vi "Set_Joint_Main_Loop.vi"(0 "X-CAN in":refnum<class "X-CAN.lvclass">, 1 "Actual position":T1(array[cluster]) {"Error Code" format="%b"; "ID" format="%x"}, 2 "Motor enabled?":bool[](array[boolean]), 5 "Reset?":bool[](array[boolean]), 7 "Desired position":u16[](array[numeric]) format="%x", 9 "Current position":u16[](array[numeric]) format="%x", 11 "error in (no error)":errorcluster, 12 "Speed":u16[](array[numeric]) format="%x", 13 "Reset speed?":bool) -> (4 "X-CAN out":refnum<class "X-CAN.lvclass">, 6 "New position":T1(array[cluster]) {"Error Code" format="%b"; "ID" format="%x"}, 15 "error out":errorcluster)   [LabVIEW 2015]
uses:
  <vilib>/Stratom, Inc/X-CAN for myRIO (API)/X-CAN Class/X-CAN.lvclass
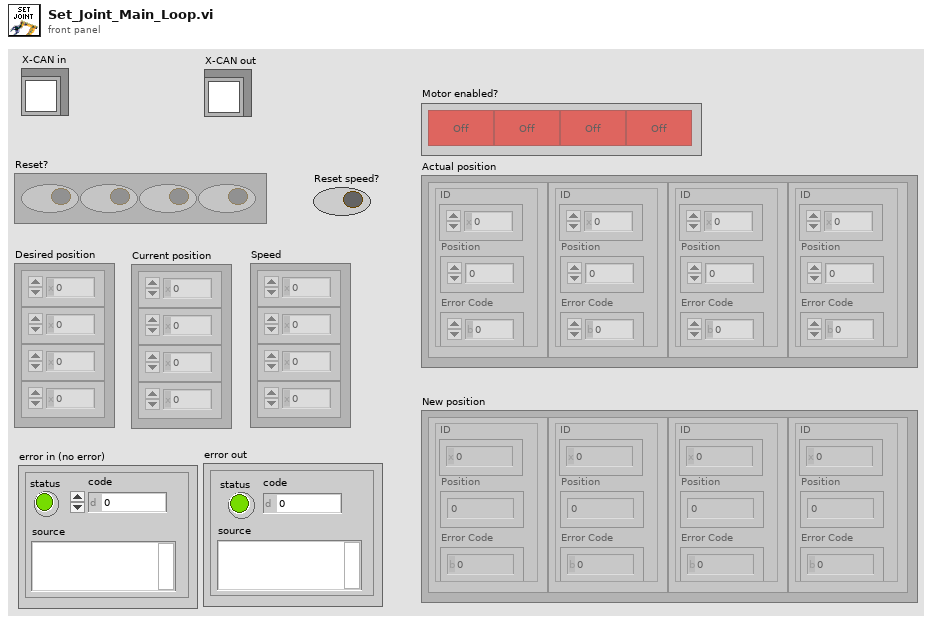
[diagram p1: front panel]
types:
  T1 = cluster{"ID":u8, "Position":u16, "Error Code":u8}[]
  T2 = typedef "X-CAN.lvclass/CANFrame.ctl" = cluster{"identifier":u32, "extended?":bool, "echo?":bool, "payload":u8[], "timestamp":timestamp}
  T3 = cluster{"Error Code":u8, "Position":u16, "ID":u8}
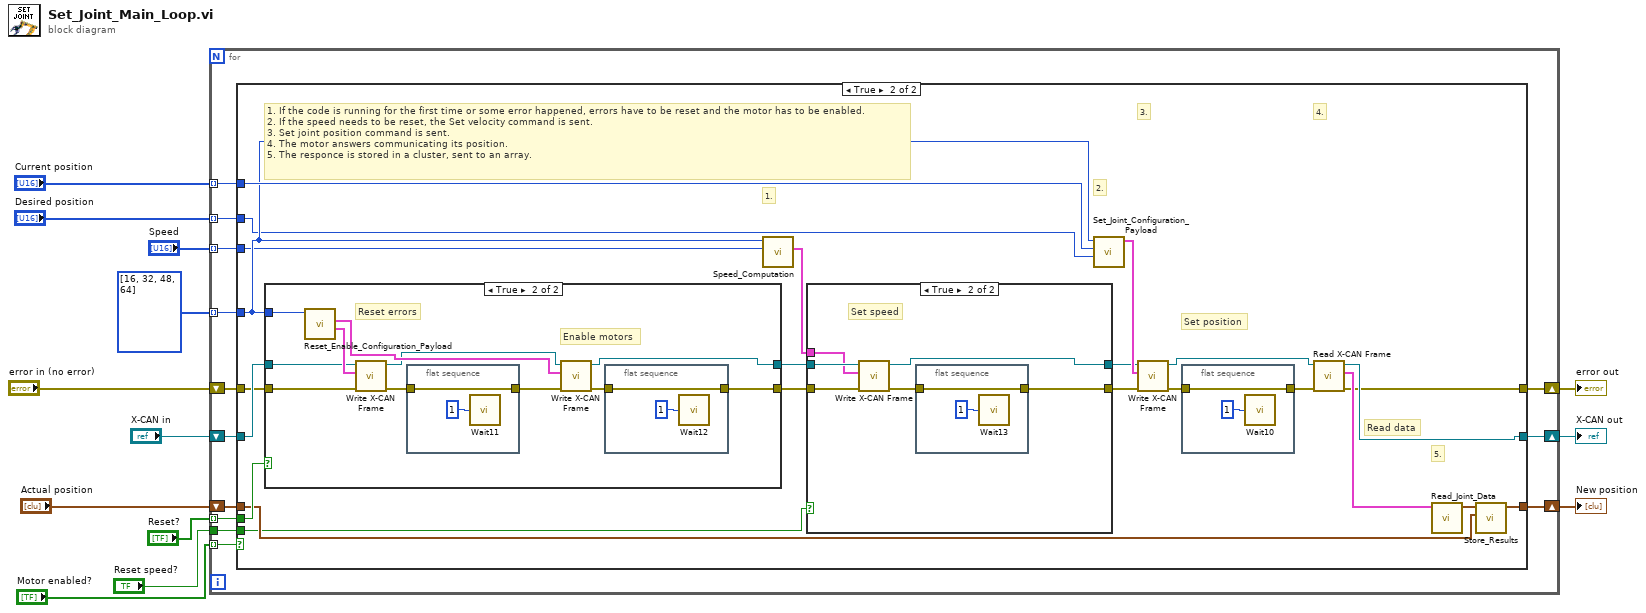
[diagram p0: block diagram]
diagram:
  n1 = for {
    shift-right: [w21] -> w10
    shift-left: "X-CAN in" -> [w26]
    shift-right: [w16] -> w11
    shift-left: "error in (no error)" -> [w25]
    tunnel: u8[] [16, 32, 48, 64] ("identifier") -> [w18] mode=indexing
    tunnel: "Reset?" -> [w24] mode=indexing
    tunnel: "Current position" -> [w20] mode=indexing
    tunnel: "Desired position" -> [w19] mode=indexing
    shift-right: [w23] -> w4
    shift-left: "Actual position" -> [w22]
    tunnel: "Speed" -> [w17] mode=indexing
    tunnel: "Motor enabled?" -> [w15] mode=indexing
    tunnel: "Reset speed?" -> [w14]
    n2 = case shown="True" w15 {
      tunnel: w26 -> [w28 w50]
      tunnel: w25 -> [w29 w49]
      tunnel: w24 -> [_ w48]
      tunnel: [w27 w47] -> w23
      tunnel: w22 -> [w27 w46]
      tunnel: [w28 w42] -> w21
      tunnel: w20 -> [_ w40]
      tunnel: w19 -> [_ w31]
      tunnel: w18 -> [_ w39]
      tunnel: w17 -> [_ w38]
      tunnel: [w29 w32] -> w16
      tunnel: w14 -> [_ w30]
      frame False {
      }
      frame True {
        # "1. If the code is running for the first time or some error happened, errors have to be reset and the motor has to be enabled.\n2. If the speed needs to be reset, the Set velocity command is sent.\n3. Set joint position command is sent.\n4. The motor answers communicating its position.\n5. The responce is stored in a cluster, sent to an array."
        # "5."
        # "4."
        # "3."
        # "2."
        # "1."
        # "Read data"
        # "Set position"
        n3 = case shown="True" w48 {
          tunnel: [w64 w69] -> w37
          tunnel: [w63 w68] -> w36
          tunnel: w50 -> [w64 w67]
          tunnel: w49 -> [w63 w66]
          tunnel: w39 -> [_ w65]
          frame False {
          }
          frame True {
            # "Enable motors"
            # "Reset errors"
            n4 = call "Reset_Enable_Configuration_Payload.vi"("identifier selection in"=w65) -> ("Reset errors command"=w71:T2, "Enable motor command"=w72:T2)  [unwired: 9 in]
            n5 = call <vilib>:"Write X-CAN Frame.vi"("error in"=w66, "CAN Frame"=w71, "X-CAN Session in"=w67) -> ("error out"=w73:errorcluster, "X-CAN Session out"=w70:refnum<class "X-CAN.lvclass">)  [unwired: 7 in]
            n6 = flat-sequence {
              tunnel: w73 -> [w78]
              tunnel: [w78] -> w75
              frame #0 {
                n7 = call "Wait11"("Count(mSec)"=u32 1 ("Tick Count(mSec)")) -> ()  [unwired: 1 out]
              }
            }
            n8 = call <vilib>:"Write X-CAN Frame.vi"("error in"=w75, "CAN Frame"=w72, "X-CAN Session in"=w70) -> ("error out"=w74:errorcluster, "X-CAN Session out"=w69:refnum<class "X-CAN.lvclass">)  [unwired: 7 in]
            n9 = flat-sequence {
              tunnel: w74 -> [w76]
              tunnel: [w76] -> w68
              frame #0 {
                n10 = call "Wait12"("Count(mSec)"=u32 1 ("Tick Count(mSec)")) -> ()  [unwired: 1 out]
              }
            }
          }
        }
        n11 = call "Speed_Computation.vi"("Speed"=w38, "identifier"=w39) -> ("output cluster"=w33:T2)  [unwired: 9 in]
        n12 = case shown="True" w30 {
          tunnel: w37 -> [w54 w60]
          tunnel: w36 -> [w53 w59]
          tunnel: [w54 w58] -> w35
          tunnel: [w53 w56] -> w34
          tunnel: w33 -> [_ w55]
          frame False {
          }
          frame True {
            # "Set speed"
            n13 = call <vilib>:"Write X-CAN Frame.vi"("error in"=w59, "CAN Frame"=w55, "X-CAN Session in"=w60) -> ("error out"=w57:errorcluster, "X-CAN Session out"=w58:refnum<class "X-CAN.lvclass">)  [unwired: 7 in]
            n14 = flat-sequence {
              tunnel: w57 -> [w61]
              tunnel: [w61] -> w56
              frame #0 {
                n15 = call "Wait13"("Count(mSec)"=u32 1 ("milliseconds to wait")) -> ()  [unwired: 1 out]
              }
            }
          }
        }
        n16 = call "Set_Joint_Configuration_Payload.vi"("Desired position"=w31, "Current position"=w40, "Identifier selection in"=w39) -> ("Set joint position command"=w52:T2)  [unwired: 8 in]
        n17 = call <vilib>:"Write X-CAN Frame.vi"("error in"=w34, "CAN Frame"=w52, "X-CAN Session in"=w35) -> ("error out"=w51:errorcluster, "X-CAN Session out"=w44:refnum<class "X-CAN.lvclass">)  [unwired: 7 in]
        n18 = flat-sequence {
          tunnel: w51 -> [w80]
          tunnel: [w80] -> w43
          frame #0 {
            n19 = call "Wait10"("Count(mSec)"=u32 1 ("milliseconds to wait")) -> ()  [unwired: 1 out]
          }
        }
        n20 = call <vilib>:"Read X-CAN Frame.vi"("error in"=w43, "X-CAN Session in"=w44) -> ("error out"=w32:errorcluster, "CAN Frame"=w41:T2, "X-CAN Session out"=w42:refnum<class "X-CAN.lvclass">)  [unwired: 7 in]
        n21 = call "Read_Joint_Data.vi"("CAN Frame"=w41) -> ("Joint Position out"=w45:T3)  [unwired: 9 in, 1 out]
        n22 = call "Store_Results.vi"("Positions in"=w46, "Joint Info"=w45) -> ("Stored positions"=w47:T1)  [unwired: 9 in]
      }
    }
  }
  "error out" <- w11
  "X-CAN out" <- w10
  "New position" <- w4
